vi "Calibration_Warning.vi"(11 "USB":tag) -> ()   [LabVIEW 2015]
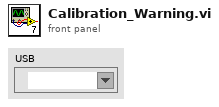
[diagram p1: front panel]
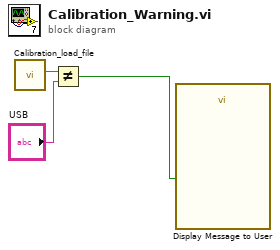
[diagram p0: block diagram]
diagram:
  n1 = call "Calibration_load_file.vi"() -> ("USB_DEV"=w2:string)  [unwired: 9 in, 2 out]
  n2 = Not Equal?(x=w2, y="USB") -> (x != y?=w1:bool)
  n3 = call "Display Message to User"("Enable"=w1) -> ()  [unwired: 9 in, 2 out]
